vi "Teleop.vi"(10 "Match Info":T1={"Autonomous Elapsed Seconds"=0.0, "TeleOp Elapsed Seconds"=0.0, "Disabled Elapsed Seconds"=0.0, "Visited Autonomous"=FALSE, "Visited TeleOp"=FALSE, "Visited Disabled"=FALSE, "Autonomous Settings"={"Autonomous Style"=enum."Independent", "VI Refnum"=refnum}}, 11 "Call Context":T2) -> ()   [LabVIEW 2019]
doc: "This VI is called for each TeleOp packet received from the DS where the robot is not disabled. It is often used to read from the joysticks and update I/O or to update setpoints for timed control loops. It should complete and return within 20 milliseconds or it may miss DS packets."
uses:
  <vilib>/Rock Robotics/WPI/DriverStation/WPI_DriverStationDerivedRobotMode.ctl
  <vilib>/Rock Robotics/WPI/DriverStation/WPI_DriverStationMatch Info.ctl
  <vilib>/Rock Robotics/WPI/Ultrasonic/WPI_UltrasonicRangeUnits.ctl
  <vilib>/Rock Robotics/WPI/Solenoid/WPI_SolenoidValue.ctl
  <vilib>/Rock Robotics/WPI/Utilities/WPI_GetSetVariantRefNum.vi
  <vilib>/Rock Robotics/Network Tables/NT Write Boolean Array.vi
  <vilib>/Rock Robotics/Network Tables/NT Write Numeric Array.vi
  <vilib>/Rock Robotics/Network Tables/NT Read Boolean.vi
  <vilib>/Rock Robotics/Network Tables/NT Read Number.vi
  <vilib>/Rock Robotics/WPI/Solenoid/WPI_SolenoidSetEnum.vi
  <vilib>/Rock Robotics/WPI/Ultrasonic/WPI_SonarSRF04DigitalRefNum Registry Get.vi
  <vilib>/Rock Robotics/WPI/Ultrasonic/WPI_SonarSRF04DigitalGetRange.vi
panel:
  out "Numeric":dbl
  out "Sample Slider 0":dbl(slide) scale=0.0..5.0
  out "Sample Boolean 1":bool
  out "Sample Boolean 0":bool
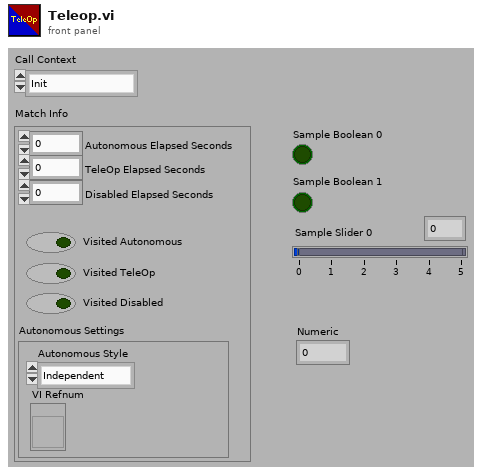
[diagram p1: front panel]
types:
  T1 = typedef "WPI_DriverStationMatch Info.ctl" = cluster{"Autonomous Elapsed Seconds":dbl, "TeleOp Elapsed Seconds":dbl, "Disabled Elapsed Seconds":dbl, "Visited Autonomous":bool, "Visited TeleOp":bool, "Visited Disabled":bool, "Autonomous Settings":cluster{"Autonomous Style":enum16{"Iterative", "Independent"}, "VI Refnum":refnum<vi>}}
  T2 = typedef "WPI_DriverStationDerivedRobotMode.ctl" = enum16{"Init", "Execute", "Stop"}
  T3 = typedef "WPI_UltrasonicRangeUnits.ctl" = enum16{"inches", "mm"}
  T4 = typedef "WPI_RobotDriveDevRef.ctl" = cluster{"DevStatus":errorcluster, "Motors[]":T5[], "Square Inputs":bool, "Max Output":dbl}
  T5 = typedef "WPI_MotorControlDeviceRef.ctl" = cluster{"DeviceStatus":errorcluster, "Type":T6, "PWM":cluster{"PWM Channel":T7, "DeadBand":T8}, "CAN":cluster{"Device Number":u8, "SetOutput VI Ref":variant, "GetOutput VI Ref":variant, "Enable VI Ref":variant, "Disable VI Ref":variant, "Data":variant}, "Invert":bool, "DIO PWM":cluster{"PWM \"Enable\" Channel":T7, "DIOChannel":T9, "PWM Rate":dbl}}
  T6 = typedef "WPI_MotorControlType.ctl" = enum16{"PWM", "CAN", "DIO PWM"}
  T7 = typedef "FPGA_DIOPWMChannel.ctl" = enum8{"PWM 0", "PWM 1", "PWM 2", "PWM 3", "PWM 4", "PWM 5", "PWM 6", "PWM 7", "PWM 8", "PWM 9", "PWM MXP 0", "PWM MXP 1", "PWM MXP 2", "PWM MXP 3", "PWM MXP 4", "PWM MXP 5", "PWM MXP 6", "PWM MXP 7", "PWM MXP 8", "PWM MXP 9", "Invalid"}
  T8 = typedef "WPI_PWMDeadband.ctl" = cluster{"Name":string, "maxPositivePwm":i32, "minPositivePwm":i32, "centerPwm":i32, "maxNegativePwm":i32, "minNegativePwm":i32, "angularRange":u16}
  T9 = typedef "FPGA_DIOChannel.ctl" = enum8{"DIO 0", "DIO 1", "DIO 2", "DIO 3", "DIO 4", "DIO 5", "DIO 6", "DIO 7", "DIO 8", "DIO 9", "DIO MXP 0", "DIO MXP 1", "DIO MXP 2", "DIO MXP 3", "DIO MXP 4", "DIO MXP 5", "DIO MXP 6", "DIO MXP 7", "DIO MXP 8", "DIO MXP 9", "DIO MXP 10", "DIO MXP 11", "DIO MXP 12", "DIO MXP 13", "DIO MXP 14", "DIO MXP 15", "SPI Port CS1", "SPI Port CS2", "SPI Port CS3", "SPI Port MISO", "SPI Port MOSI", "Invalid"}
  T10 = typedef "WPI_JoystickDevRef.ctl" = cluster{"Device":T11}
  T11 = typedef "WPI_JoystickDeviceEnum.ctl" = enum16{"USB 0", "USB 1", "USB 2", "USB 3", "USB 4", "USB 5"}
  T12 = typedef "WPI_AnalogChannelDevRef.ctl" = cluster{"DevStatus":errorcluster, "Analog Channel":T13}
  T13 = typedef "FPGA_AIChannel.ctl" = enum8{"AI 0", "AI 1", "AI 2", "AI 3", "AI MXP 0", "AI MXP 1", "AI MXP 2", "AI MXP 3", "Invalid"}
  T14 = typedef "WPI_SolenoidValue.ctl" = enum16{"Off", "On", "Forward", "Reverse"}
  T15 = typedef "WPI_SolenoidDevRef.ctl" = cluster{"DevStatus":errorcluster, "Pneumatics Control Module":u8, "Forward Solenoid Channel":T16, "Reverse Solenoid Channel":T16}
  T16 = typedef "WPI_SolenoidChannel.ctl" = enum8{"Solenoid 0", "Solenoid 1", "Solenoid 2", "Solenoid 3", "Solenoid 4", "Solenoid 5", "Solenoid 6", "Solenoid 7", "Invalid"}
  T17 = typedef "WPI_PWMDeviceRef.ctl" = cluster{"DeviceStatus":errorcluster, "PWM Channel":T7}
  T18 = typedef "WPI_UltrasonicDeviceRef.ctl" = cluster{"DevStatus":errorcluster, "Ping Channel":T9, "Echo Channel":T9, "CntIndex":T19}
  T19 = typedef "FPGA_CounterCtrSystemIndex.ctl" = enum8{"Ctr 0", "Ctr 1", "Ctr 2", "Ctr 3", "Ctr 4", "Ctr 5", "Ctr 6", "Ctr 7", "Invalid"}
  T20 = typedef "WPI_CompressorDevRef.ctl" = cluster{"DevStatus":errorcluster, "Pneumatics Control Module":u8}
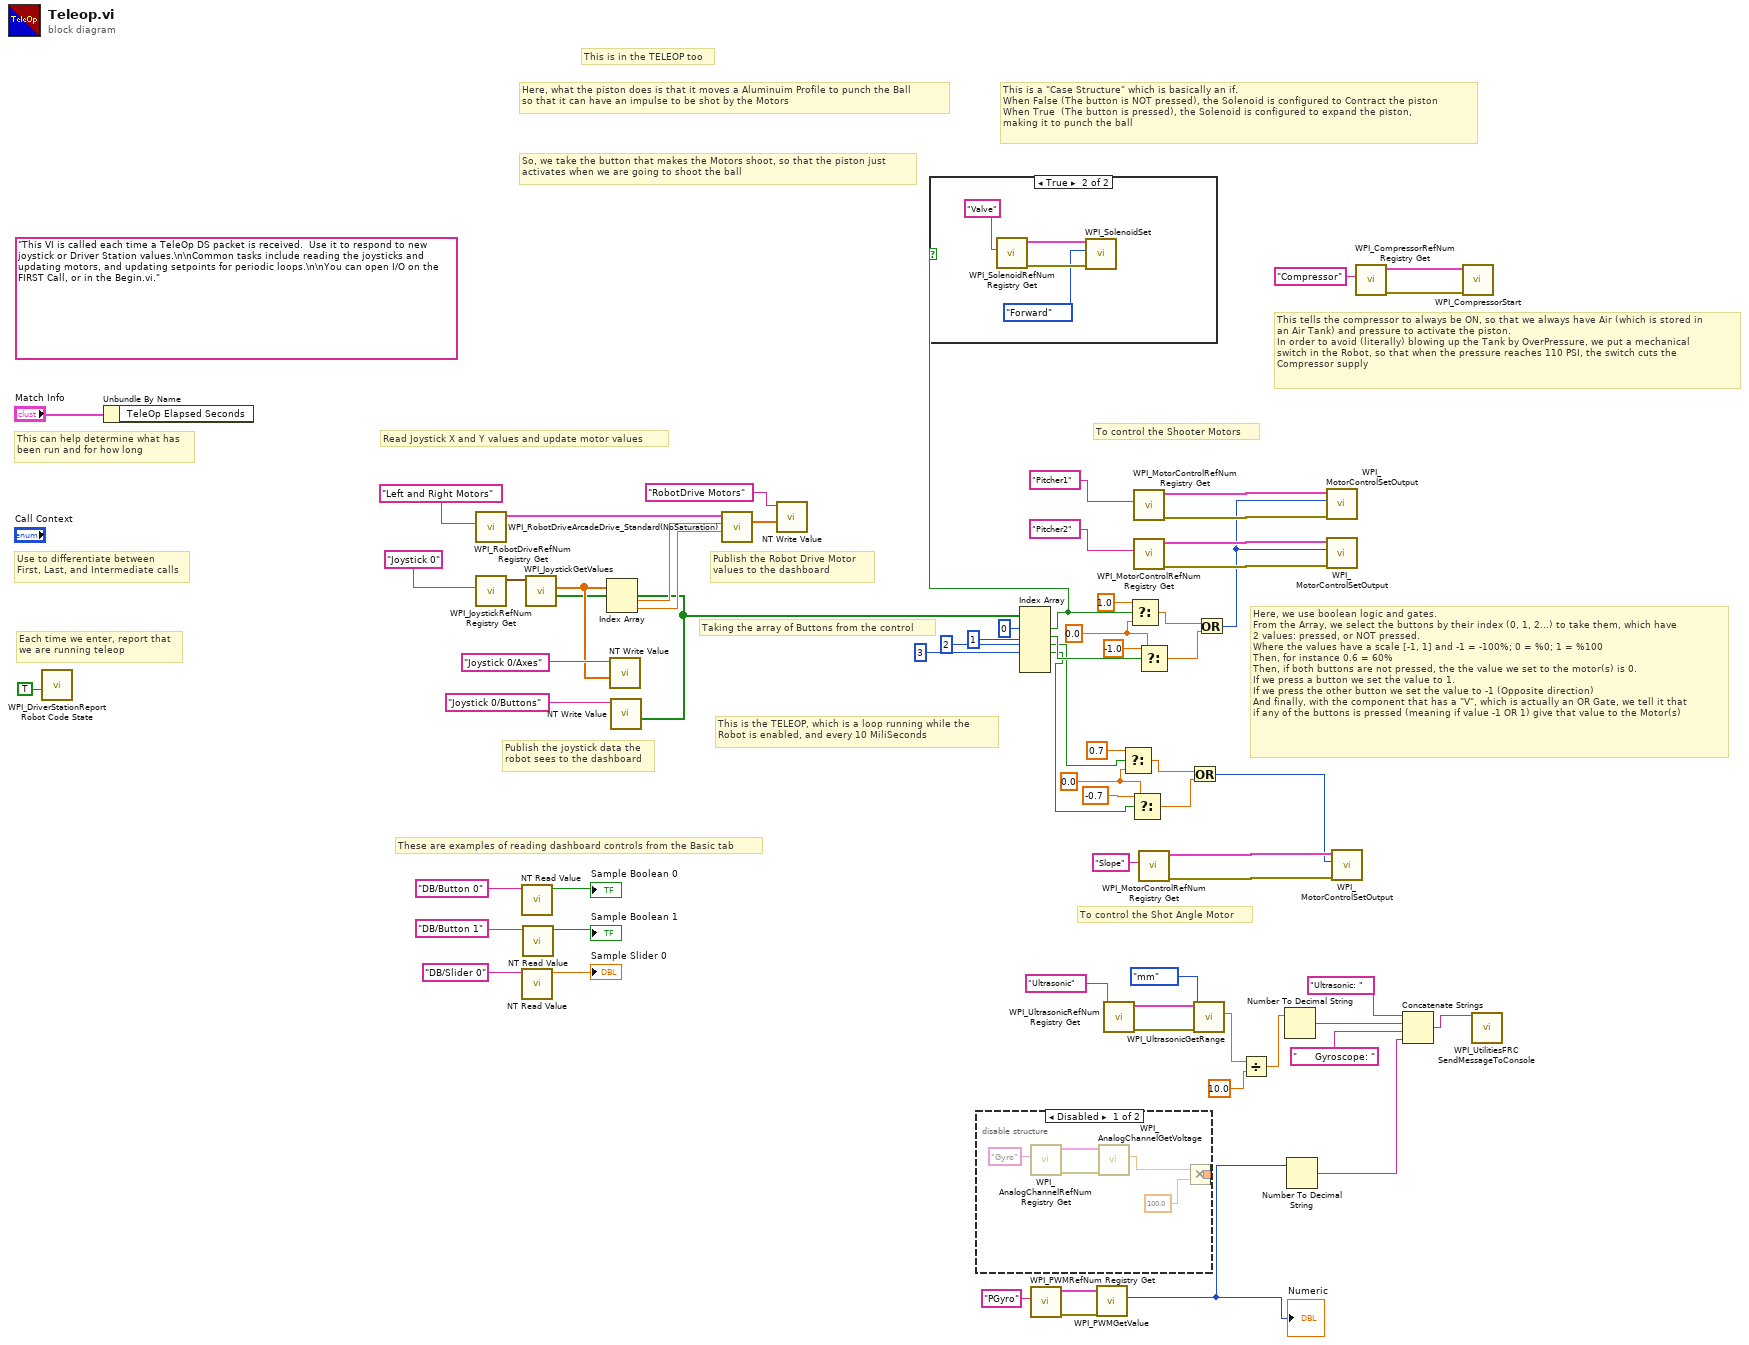
[diagram p0: block diagram]
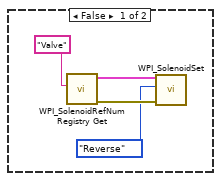
[diagram p3: hidden frame]
diagram:
  w30 = 0.0 ("f")
  w42 = 0.0 ("f")
  (unwired) "This VI is called each time a TeleOp DS packet is received.  Use it to respond to new joystick or Driver Station values.\n\nCommon tasks include reading the joysticks and updating motors, and updating setpoints for periodic loops.\n\nYou can open I/O on the FIRST Call, or in the Begin.vi."
  # "This tells the compressor to always be ON, so that we always have Air (which is stored in\nan Air Tank) and pressure to activate the piston.\nIn order to avoid (literally) blowing up the Tank by OverPressure, we put a mechanical\nswitch in the Robot, so that when the pressure reaches 110 PSI, the switch cuts the \nCompressor supply"
  # "This is a \"Case Structure\" which is basically an if.\nWhen False (The button is NOT pressed), the Solenoid is configured to Contract the piston\nWhen True  (The button is pressed), the Solenoid is configured to expand the piston,\nmaking it to punch the ball"
  # "So, we take the button that makes the Motors shoot, so that the piston just\nactivates when we are going to shoot the ball"
  # "This is in the TELEOP too"
  # "Here, what the piston does is that it moves a Aluminuim Profile to punch the Ball\nso that it can have an impulse to be shot by the Motors"
  # "This is the TELEOP, which is a loop running while the \nRobot is enabled, and every 10 MiliSeconds"
  # "To control the Shooter Motors"
  # "To control the Shot Angle Motor"
  # "Here, we use boolean logic and gates.\nFrom the Array, we select the buttons by their index (0, 1, 2...) to take them, which have\n2 values: pressed, or NOT pressed.\nWhere the values have a scale [-1, 1] and -1 = -100%; 0 = %0; 1 = %100\nThen, for instance 0.6 = 60%\nThen, if both buttons are not pressed, the the value we set to the motor(s) is 0.\nIf we press a button we set the value to 1.\nIf we press the other button we set the value to -1 (Opposite direction)\nAnd finally, with the component that has a \"V\", which is actually an OR Gate, we tell it that\nif any of the buttons is pressed (meaning if value -1 OR 1) give that value to the Motor(s)"
  # "Taking the array of Buttons from the control"
  # "These are examples of reading dashboard controls from the Basic tab"
  # "Publish the Robot Drive Motor\nvalues to the dashboard"
  # "Publish the joystick data the\nrobot sees to the dashboard"
  # "Each time we enter, report that\nwe are running teleop"
  # "Use to differentiate between\nFirst, Last, and Intermediate calls"
  # "This can help determine what has\nbeen run and for how long"
  # "Read Joystick X and Y values and update motor values"
  n1 = call <vilib>:"WPI_DriverStationReport Robot Code State.vi"("TeleOp"=TRUE ("Autonomous")) -> ()  [unwired: 10 in, 1 out]
  n2 = Unbundle By Name("Match Info") -> ()  [unwired: 1 out]
  n3 = call <vilib>:"WPI_RobotDriveRefNum Registry Get.vi"("refnum name"="Left and Right Motors") -> ("RobotDriveDevRef"=w66:T4)  [unwired: 1 in, 9 out]
  n4 = call <vilib>:"WPI_JoystickRefNum Registry Get.vi"("refnum name"="Joystick 0") -> ("JoystickDevRef"=w63:T10)  [unwired: 1 in, 9 out]
  n5 = call-poly <vilib>:"NT Read Value.vi"("Name"="DB/Button 0" ("refnum name")) -> ("Boolean"=→"Sample Boolean 0":bool)  [unwired: 9 in, 1 out]
  n6 = call-poly <vilib>:"NT Read Value.vi"("Name"="DB/Slider 0" ("refnum name")) -> ("Numeric"=→"Sample Slider 0":dbl)  [unwired: 9 in, 1 out]
  n7 = call-poly <vilib>:"NT Read Value.vi"("Name"="DB/Button 1" ("refnum name")) -> ("Boolean"=→"Sample Boolean 1":bool)  [unwired: 9 in, 1 out]
  n8 = call <vilib>:"WPI_JoystickGetValues.vi"("JoystickDevRef"=w63) -> ("Buttons"=w49:bool[], "Axes"=w58:dbl[])  [unwired: 6 in, 3 out]
  n9 = Index Array(array=w58) -> (element #1=w65:dbl, element #2=w61:dbl)  [unwired: 2 in]
  n10 = call-poly <vilib>:"NT Write Value.vi"("Numeric Array"=w58, "Name"="Joystick 0/Axes") -> ()  [unwired: 9 in, 1 out]
  n11 = call-poly <vilib>:"NT Write Value.vi"("Boolean Array"=w49, "Name"="Joystick 0/Buttons") -> ()  [unwired: 9 in, 1 out]
  n12 = call <vilib>:"WPI_RobotDriveArcadeDrive_Standard(NoSaturation).vi"("Y axis value"=w61, "X axis value"=w65, "RobotDriveDevRef"=w66) -> ("Motor Values"=w51:dbl[])  [unwired: 1 in, 7 out]
  n13 = call-poly <vilib>:"NT Write Value.vi"("Numeric Array"=w51, "Name"="RobotDrive Motors") -> ()  [unwired: 9 in, 1 out]
  n14 = disable-structure shown="Disabled" {
    disable-tunnel: [w70 _] -> _
    frame Disabled {
      n15 = call <vilib>:"WPI_AnalogChannelRefNum Registry Get.vi"("refnum name"="Gyro") -> ("error out"=w73:errorcluster, "AIDeviceRef"=w74:T12)  [unwired: 9 in]
      n16 = call <vilib>:"WPI_AnalogChannelGetVoltage.vi"("error in (no error)"=w73, "AIDeviceRef"=w74) -> ("Voltage"=w71:dbl)  [unwired: 7 in, 2 out]
      n17 = Multiply(x=w71, y=100.0) -> (x*y=w70:dbl)
    }
    frame Enabled {
    }
  }
  n18 = Index Array(array=w49, index #1=0 ("index"), index #2=1 ("index"), index #3=2 ("index"), index #4=3 ("index")) -> (element #1=w17:bool, element #2=w44:bool, element #3=w26:bool, element #4=w25:bool)  [unwired: 2 in, 2 out]
  n19 = case shown="True" w17 {
    frame False {
      n20 = call <vilib>:"WPI_SolenoidRefNum Registry Get.vi"("refnum name"="Valve") -> ("error out"=w77:errorcluster, "SolenoidDevRef"=w78:T15)  [unwired: 9 in]
      n21 = call-poly <vilib>:"WPI_SolenoidSet.vi"("error in (no error)"=w77, "Value"=WPI_SolenoidValue."Reverse", "SolenoidDevRef"=w78) -> ()  [unwired: 7 in, 2 out]
    }
    frame True {
      n22 = call <vilib>:"WPI_SolenoidRefNum Registry Get.vi"("refnum name"="Valve") -> ("error out"=w81:errorcluster, "SolenoidDevRef"=w82:T15)  [unwired: 9 in]
      n23 = call-poly <vilib>:"WPI_SolenoidSet.vi"("error in (no error)"=w81, "Value"=WPI_SolenoidValue."Forward", "SolenoidDevRef"=w82) -> ()  [unwired: 7 in, 2 out]
    }
  }
  n24 = call <vilib>:"WPI_PWMRefNum Registry Get.vi"("refnum name"="PGyro") -> ("error out"=w3:errorcluster, "PWMDeviceRef"=w4:T17)  [unwired: 9 in]
  n25 = call <vilib>:"WPI_PWMGetValue.vi"("error in (no error)"=w3, "PWMDeviceRef"=w4) -> ("Value"=w1:u16)  [unwired: 7 in, 2 out]
  "Numeric" <- w1
  n26 = call-poly <vilib>:"WPI_UltrasonicRefNum Registry Get.vi"("refnum name"="Ultrasonic") -> ("error out"=w15:errorcluster, "SonarSRF04DevRef"=w16:T18)  [unwired: 9 in]
  n27 = Select(t=0.7, s=w26, f=w30) -> (s? t:f=w28:dbl)
  n28 = Select(t=1.0, s=w17, f=w42) -> (s? t:f=w40:dbl)
  n29 = Select(t=-0.7, s=w25, f=w30) -> (s? t:f=w27:dbl)
  n30 = call <vilib>:"WPI_MotorControlRefNum Registry Get.vi"("refnum name"="Pitcher1") -> ("error out"=w37:errorcluster, "MotorControlDevRef"=w38:T5)  [unwired: 9 in]
  n31 = call <vilib>:"WPI_MotorControlRefNum Registry Get.vi"("refnum name"="Pitcher2") -> ("error out"=w34:errorcluster, "MotorControlDevRef"=w35:T5)  [unwired: 9 in]
  n32 = Select(t=-1.0, s=w44, f=w42) -> (s? t:f=w39:dbl)
  n33 = call <vilib>:"WPI_MotorControlRefNum Registry Get.vi"("refnum name"="Slope") -> ("error out"=w23:errorcluster, "MotorControlDevRef"=w24:T5)  [unwired: 9 in]
  n34 = Or(x=w28, y=w27) -> (x .or. y?=w21:i32)
  n35 = call-poly <vilib>:"WPI_UltrasonicGetRange.vi"("error in (no error)"=w15, "Range Units"=WPI_UltrasonicRangeUnits."mm", "SonarSRF04DevRef"=w16) -> ("Distance"=w12:dbl)  [unwired: 6 in, 2 out]
  n36 = Or(x=w40, y=w39) -> (x .or. y?=w32:i32)
  n37 = Divide(x=w12, y=10.0) -> (x/y=w10:dbl)
  n38 = Number To Decimal String(number=w10) -> (decimal integer string=w8:string)  [unwired: 1 in]
  n39 = Number To Decimal String(number=w1) -> (decimal integer string=w6:string)  [unwired: 1 in]
  n40 = call <vilib>:"WPI_MotorControlSetOutput.vi"("error in (no error)"=w37, "Output"=w32, "MotorControlDevRef"=w38) -> ()  [unwired: 6 in, 3 out]
  n41 = call <vilib>:"WPI_MotorControlSetOutput.vi"("error in (no error)"=w34, "Output"=w32, "MotorControlDevRef"=w35) -> ()  [unwired: 6 in, 3 out]
  n42 = call <vilib>:"WPI_MotorControlSetOutput.vi"("error in (no error)"=w23, "Output"=w21, "MotorControlDevRef"=w24) -> ()  [unwired: 6 in, 3 out]
  n43 = call <vilib>:"WPI_CompressorRefNum Registry Get.vi"("refnum name"="Compressor") -> ("error out"=w19:errorcluster, "CompressorDevRef"=w20:T20)  [unwired: 9 in]
  n44 = Concatenate Strings("Ultrasonic: " ("string"), w8, "      Gyroscope: " ("string"), w6) -> (w5:string)
  n45 = call <vilib>:"WPI_CompressorStart.vi"("error in (no error)"=w19, "CompressorDevRef"=w20) -> ()  [unwired: 8 in, 2 out]
  n46 = call <vilib>:"WPI_UtilitiesFRC SendMessageToConsole.vi"("Message"=w5) -> ()  [unwired: 14 in, 1 out]
